vi "TDMS_write.vi"() -> ()   [LabVIEW 2011]
panel:
  out "error out 2":errorcluster
  in  "stop 2":bool
  out "error out":errorcluster
  in  "stop":bool
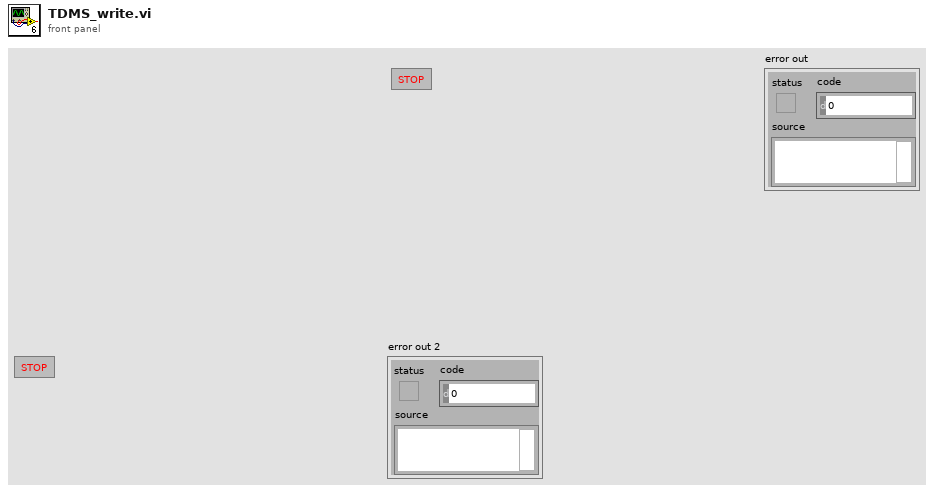
[diagram p1: front panel]
types:
  T1 = enum16{"open", "open or create", "create or replace", "create", "open (read-only)"}
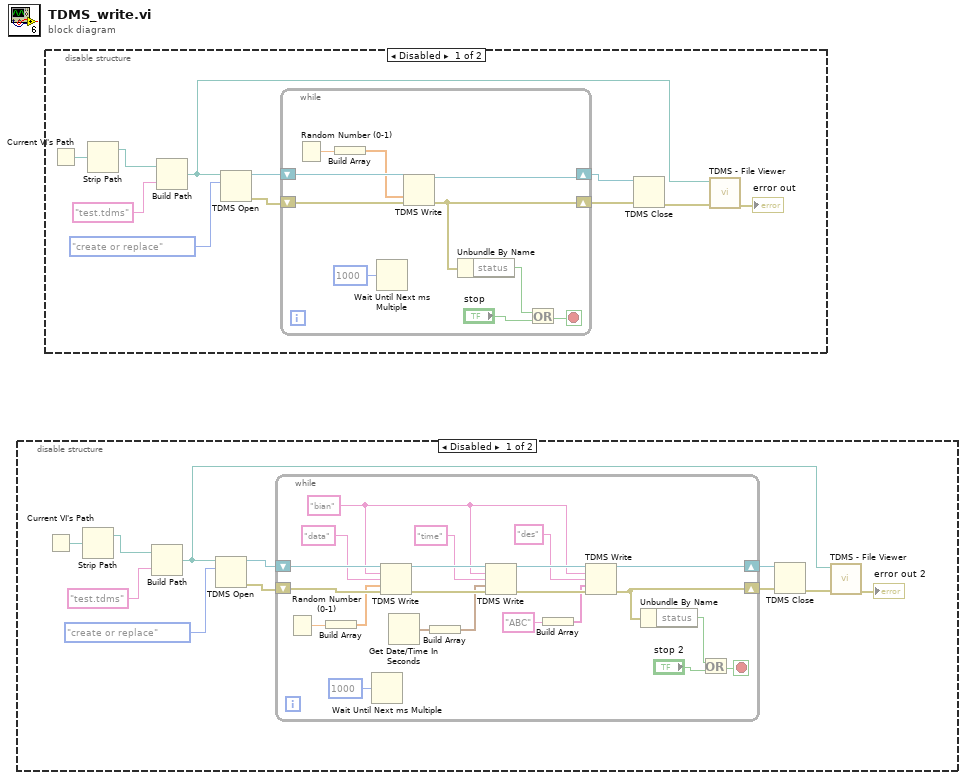
[diagram p0: block diagram]
diagram:
  n1 = disable-structure shown="Disabled" {
    frame Disabled {
      n2 = Current VI's Path() -> (path=w9:path)
      n3 = Strip Path(path=w9) -> (stripped path=w8:path)  [unwired: 1 out]
      n4 = Build Path(base path=w8, name or relative path="test.tdms") -> (appended path=w5:path)
      n5 = TDMS Open(10:T1."create or replace" ("operation (0:open)"), 11:w5) -> (0:w10:errorcluster, 3:w11:refnum<k34>)  [unwired: 4 in]
      n6 = while {
        shift-right: [w21] -> w4
        shift-left: w11 -> [w33]
        shift-right: [w20] -> w3
        shift-left: w10 -> [w32]
        stop <- w29 stop-if-true
        w19 = "bian" ("group name in (Untitled)")
        n7 = Random Number (0-1)() -> (number: 0 to 1=w31:dbl)
        n8 = Build Array(w31) -> (w30:dbl[])
        n9 = Wait Until Next ms Multiple(millisecond multiple=u32 1000) -> ()  [unwired: 1 out]
        n10 = TDMS Write(0:w33, 5:w19, 7:"data" ("group name in (Untitled)"), 9:w30, 11:w32) -> (4:w25:refnum<k34>, 15:w24:errorcluster)  [unwired: 1 in, 2 out]
        n11 = Get Date/Time In Seconds() -> (seconds since 1Jan1904=w18:timestamp)
        n12 = Build Array(w18) -> (w17:timestamp[])
        n13 = TDMS Write(0:w25, 5:w19, 7:"time" ("group name in (Untitled)"), 9:w17, 11:w24) -> (4:w22:refnum<k34>, 15:w23:errorcluster)  [unwired: 1 in, 2 out]
        n14 = Build Array("ABC" ("group name in (Untitled)")) -> (w15:string[])
        n15 = TDMS Write(0:w22, 5:w19, 7:"des" ("group name in (Untitled)"), 9:w15, 11:w23) -> (4:w21:refnum<k34>, 15:w20:errorcluster)  [unwired: 1 in, 2 out]
        n16 = Unbundle By Name(w20) -> ("status"=w27:bool)
        n17 = Or(x=w27, y="stop 2") -> (x .or. y?=w29:bool)
      }
      n18 = TDMS Close(8:w3, 11:w4) -> (0:w2:errorcluster)  [unwired: 1 out]
      n19 = call <vilib>:"TDMS - File Viewer.vi"("error in (no error)"=w2, "file path"=w5) -> ("error out"=→"error out 2":errorcluster)  [unwired: 4 in, 1 out]
    }
    frame Enabled {
    }
  }
  n20 = disable-structure shown="Disabled" {
    frame Disabled {
      n21 = Current VI's Path() -> (path=w42:path)
      n22 = Strip Path(path=w42) -> (stripped path=w41:path)  [unwired: 1 out]
      n23 = Build Path(base path=w41, name or relative path="test.tdms") -> (appended path=w38:path)
      n24 = TDMS Open(10:T1."create or replace" ("operation (0:open)"), 11:w38) -> (0:w43:errorcluster, 3:w44:refnum<k34>)  [unwired: 4 in]
      n25 = while {
        shift-right: [w50] -> w37
        shift-left: w44 -> [w54]
        shift-right: [w47] -> w36
        shift-left: w43 -> [w53]
        stop <- w49 stop-if-true
        n26 = Random Number (0-1)() -> (number: 0 to 1=w52:dbl)
        n27 = Build Array(w52) -> (w51:dbl[])
        n28 = Wait Until Next ms Multiple(millisecond multiple=u32 1000) -> ()  [unwired: 1 out]
        n29 = TDMS Write(0:w54, 9:w51, 11:w53) -> (4:w50:refnum<k34>, 15:w47:errorcluster)  [unwired: 3 in, 2 out]
        n30 = Unbundle By Name(w47) -> ("status"=w46:bool)
        n31 = Or(x=w46, y="stop") -> (x .or. y?=w49:bool)
      }
      n32 = TDMS Close(8:w36, 11:w37) -> (0:w35:errorcluster)  [unwired: 1 out]
      n33 = call <vilib>:"TDMS - File Viewer.vi"("error in (no error)"=w35, "file path"=w38) -> ("error out"=→"error out":errorcluster)  [unwired: 4 in, 1 out]
    }
    frame Enabled {
    }
  }
